vi "Program Set Point.vi"(8 "error in (no error)":errorcluster, 10 "Set Point":dbl, 11 "Neocera in":refnum<class "Neocera.lvclass">) -> (0 "error out":errorcluster, 3 "Neocera out":refnum<class "Neocera.lvclass">)   [LabVIEW 2015, in "Neocera.lvclass"]
uses:
  Neocera.lvclass
  Mag Lab Hardware.lvclass/Mag Lab Hardware.ctl
  Mag Lab Hardware.lvclass
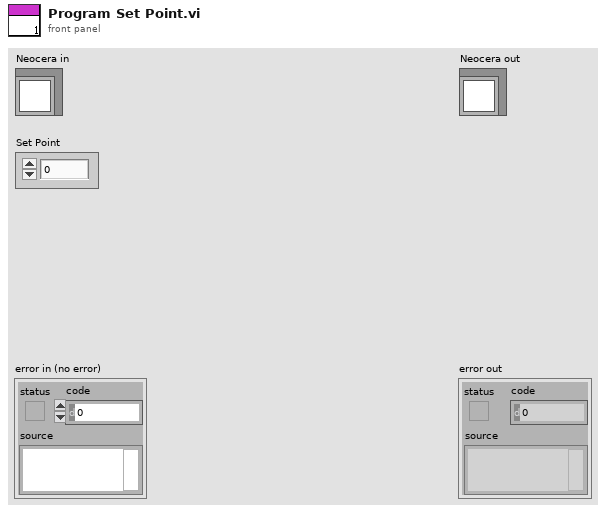
[diagram p1: front panel]
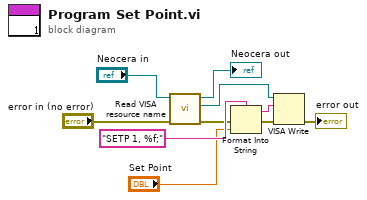
[diagram p0: block diagram]
diagram:
  n1 = call "Read VISA resource name.vi"("error in (no error)"="error in (no error)", "Mag Lab Hardware in"="Neocera in") -> ("error out"=w2:errorcluster, "VISA resource name"=w3:refnum<visa-resource-name>, "Mag Lab Hardware out"=→"Neocera out":refnum<class "Neocera.lvclass">)  [unwired: 7 in]
  n2 = Format Into String(format string="SETP 1, %f;", error in=w2, "Set Point") -> (resulting string=w7:string, error out=w5:errorcluster)  [unwired: 1 in]
  n3 = VISA Write(VISA resource name=w3, write buffer=w7, error in (no error)=w5) -> (error out=→"error out":errorcluster)  [unwired: 2 out]
